vi "To String Test.vi"() -> (0 "error out":errorcluster)   [LabVIEW 2014, in "Missing Plugin tests.lvlib"]
doc: "Test functionality of \"Missing Plugin configuration.to string\" function. VI should throw error when run."
uses:
  Missing Plugin tests.lvlib
  module/configuration/Missing Plugin configuration.lvclass
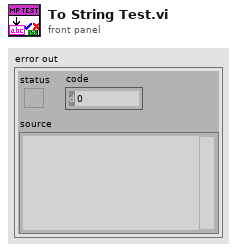
[diagram p1: front panel]
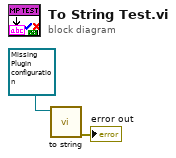
[diagram p0: block diagram]
diagram:
  n1 = call-dynamic "to string.vi"("Missing Plugin configuration in"=refnum<class "Missing Plugin configuration.lvclass"> refnum) -> ("error out"=→"error out":errorcluster)  [unwired: 7 in, 3 out]
